vi "ReadValByRef.vi"   [LabVIEW 2019]
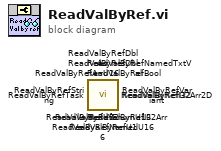
[diagram p0: block diagram]
diagram:
  n1 = call <userlib>:"ReadValByRefEnumU16.vi"() -> ()  [unwired: 12 in, 4 out]
  n2 = call <userlib>:"ReadValByRefNamedTxtVal.vi"() -> ()  [unwired: 14 in, 2 out]
  n3 = call <userlib>:"ReadValByRefTask.vi"() -> ()  [unwired: 14 in, 2 out]
  n4 = call <userlib>:"ReadValByRefI32Arr2D.vi"() -> ()  [unwired: 14 in, 2 out]
  n5 = call <userlib>:"ReadValByRefNamedU16.vi"() -> ()  [unwired: 12 in, 4 out]
  n6 = call <userlib>:"ReadValByRefArrU16.vi"() -> ()  [unwired: 14 in, 2 out]
  n7 = call <userlib>:"ReadValByRefDblArr.vi"() -> ()  [unwired: 14 in, 2 out]
  n8 = call <userlib>:"ReadValByRefI32Arr.vi"() -> ()  [unwired: 14 in, 2 out]
  n9 = call <userlib>:"ReadValByRefString.vi"() -> ()  [unwired: 14 in, 2 out]
  n10 = call <userlib>:"ReadValByRefI32.vi"() -> ()  [unwired: 14 in, 2 out]
  n11 = call <userlib>:"ReadValByRefU16.vi"() -> ()  [unwired: 14 in, 2 out]
  n12 = call <userlib>:"ReadValByRefU32.vi"() -> ()  [unwired: 14 in, 2 out]
  n13 = call <userlib>:"ReadValByRefBool.vi"() -> ()  [unwired: 14 in, 2 out]
  n14 = call <userlib>:"ReadValByRefDbl.vi"() -> ()  [unwired: 14 in, 2 out]
  n15 = call <userlib>:"ReadValByRefVariant.vi"() -> ()  [unwired: 14 in, 2 out]
